vi "default_headers.vi"(8 "error in (no error)":errorcluster, 10 "Headers":refnum<class "Headers.lvclass">, 11 "ClientBuilder in":refnum<class "ClientBuilder.lvclass">) -> (0 "error out":errorcluster, 2 "success":bool, 3 "ClientBuilder out":refnum<class "ClientBuilder.lvclass">)   [LabVIEW 2020, in "reqwest.lvlib" / "ClientBuilder.lvclass"]
uses:
  ClientBuilder.lvclass
  ClientBuilder.lvclass/ClientBuilder.ctl
  Headers/Headers.lvclass
  lv_reqwest_64.dll
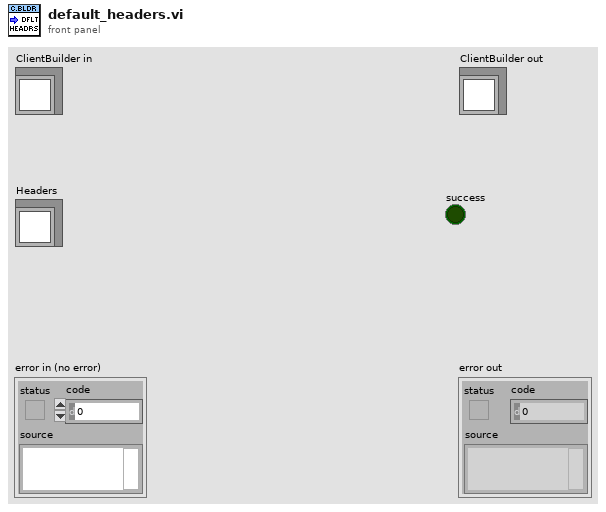
[diagram p1: front panel]
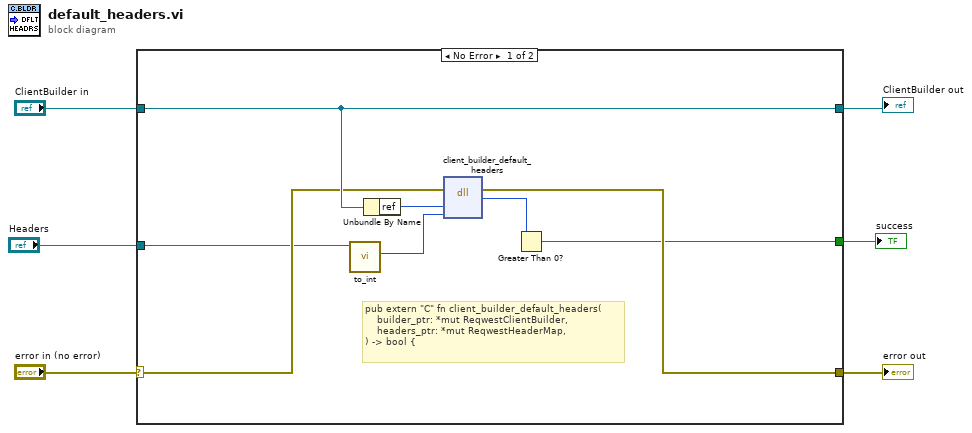
[diagram p0: block diagram]
diagram:
  n1 = case shown="No Error" "error in (no error)" {
    selector: "error in (no error)" -> [w11 w15]
    tunnel: "ClientBuilder in" -> [w12 w16]
    tunnel: [w14 w15] -> w3
    tunnel: [w12 w16] -> w4
    tunnel: "Headers" -> [w8 _]
    tunnel: [w9 _] -> w1
    frame No Error {
      # "pub extern \"C\" fn client_builder_default_headers(\n    builder_ptr: *mut ReqwestClientBuilder,\n    headers_ptr: *mut ReqwestHeaderMap,\n) -> bool {"
      n2 = call "to_int.vi"("Headers in"=w8) -> ("ref"=w7:u64)  [unwired: 10 in]
      n3 = Unbundle By Name(w12) -> ("ref"=w13:u64)
      n4 = dll-call lib="C:/Projects/reqwest-rs-labview/lv_src/lv_reqwest_64.dll" fn="client_builder_default_headers"(error in=w11, "client_builder_ref"=w13, "headers_ref"=w7) -> (error out=w14:errorcluster, "success"=w10:u8)  [unwired: 4 in, 1 out]
      n5 = Greater Than 0?(x=w10) -> (x > 0?=w9:bool)
    }
    frame Error {
    }
  }
  "error out" <- w3
  "ClientBuilder out" <- w4
  "success" <- w1
